vi "calc_sinlge JumpWaveform_v0.03.vi"(0 "New input cluster":T1={"Which Position to use for Experiment"=enum."Jumper Safe Position", "Start Position (N)"="", "Jump Position (m)"="", "Duration (s)"=0.0, "Delay (s)"=0.0, "Pulse Width (s)"=0.0, "Valve 1 Position"=0, "Valve 2 Position"=0, "Replicates"=0.0, "Vholding (mV)"=0.0, "Valve 3 Position"=1, "valve 1 used now?"=TRUE, "valve 2 used now?"=FALSE, "valve 3 used now? "=FALSE, "protocol Preview"=[]} {"Valve 3 Position" min=1 max=8}, 1 "Clear Waveform?":bool, 5 "Old input cluster":T1={"Which Position to use for Experiment"=enum."Jumper Safe Position", "Start Position (N)"="", "Jump Position (m)"="", "Duration (s)"=0.0, "Delay (s)"=0.0, "Pulse Width (s)"=0.0, "Valve 1 Position"=0, "Valve 2 Position"=0, "Replicates"=0.0, "Vholding (mV)"=0.0, "Valve 3 Position"=1, "valve 1 used now?"=TRUE, "valve 2 used now?"=FALSE, "valve 3 used now? "=FALSE, "protocol Preview"=[]} {"Valve 3 Position" min=1 max=8}, 7 "sample freq":i32=10000, 9 "Jump Filter Freq (Hz)":dbl=30.0, 11 "error in":errorcluster) -> (4 "output cluster":T1={"Which Position to use for Experiment"=enum."Jumper Safe Position", "Start Position (N)"="", "Jump Position (m)"="", "Duration (s)"=0.0, "Delay (s)"=0.0, "Pulse Width (s)"=0.0, "Valve 1 Position"=0, "Valve 2 Position"=0, "Replicates"=0.0, "Vholding (mV)"=0.0, "Valve 3 Position"=1, "valve 1 used now?"=TRUE, "valve 2 used now?"=FALSE, "valve 3 used now? "=FALSE, "protocol Preview"=[]} {"Valve 3 Position" min=1 max=8}, 15 "error out":errorcluster)   [LabVIEW 2019]
uses:
  <vilib>/Analysis/3filter.llb/Filter Passband Type.ctl
  <vilib>/Analysis/3filter.llb/Bessel Filter (DBL).vi
  <vilib>/Analysis/NI_AALBase.lvlib
  <vilib>/measure/NI_MABase.lvlib
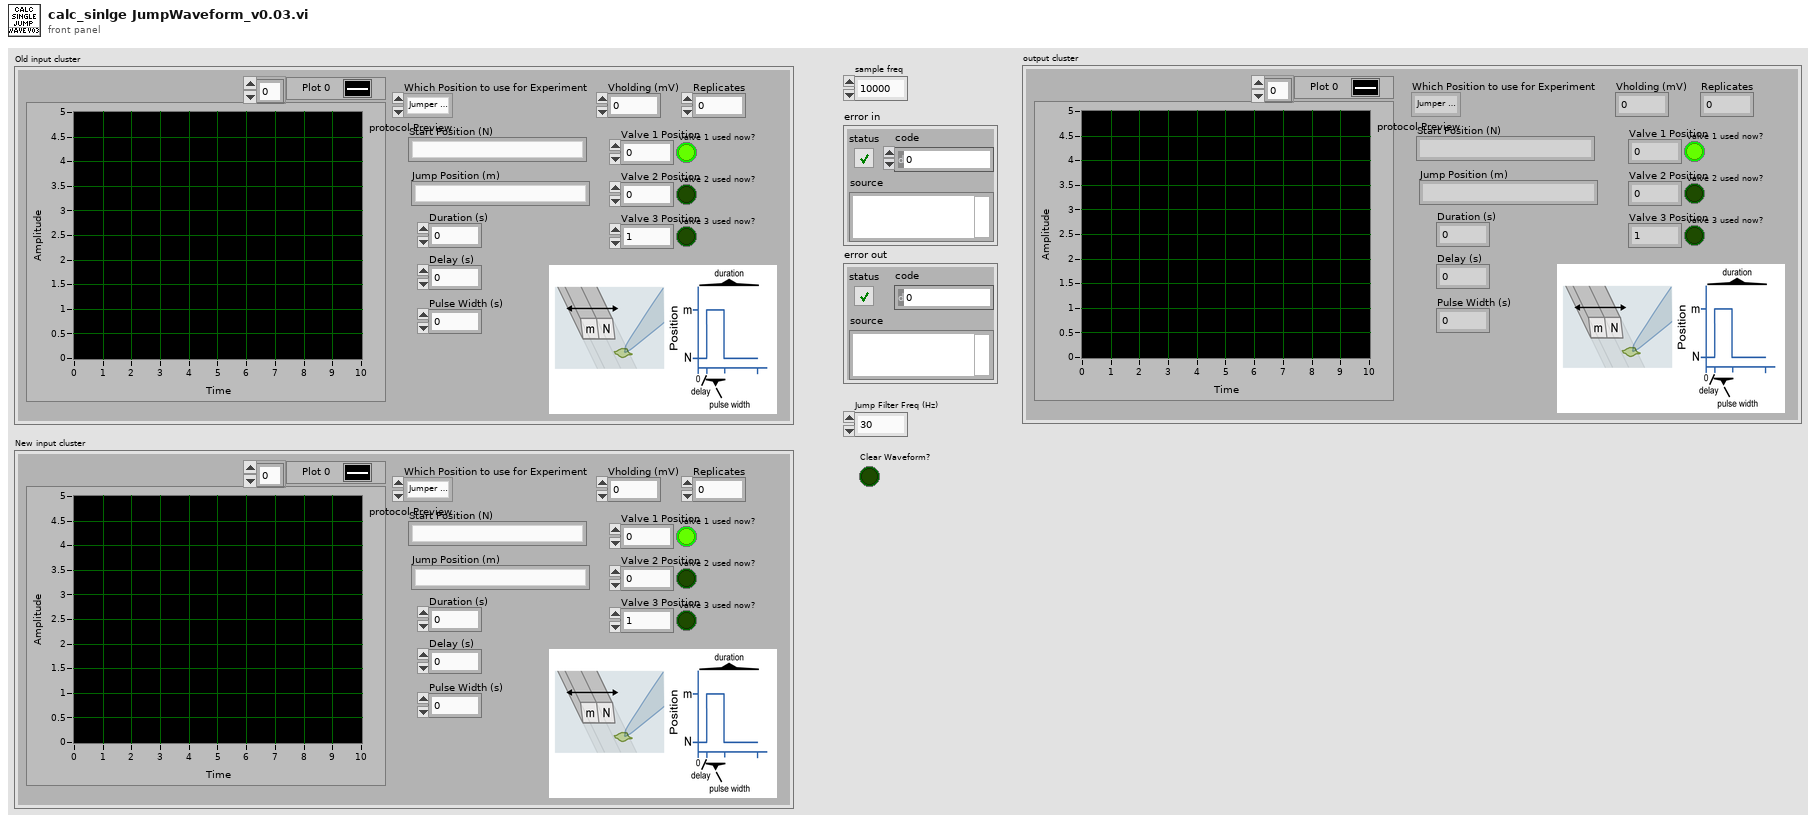
[diagram p1: front panel]
types:
  T1 = cluster{"Which Position to use for Experiment":enum16{"Jumper Safe Position", "Experiment Safe Position", "Jumper Position A", "Jumper Position B", "Jumper Position C", "Jumper Position o-A", "Jumper Position A-o", "Jumper Position A-B", "Jumper Position B-A", "Jumper Position B-C", "Jumper Position C-B", "Jumper Position C-o", "Jumper Position o-C", "Don't Move"}, "Start Position (N)":string, "Jump Position (m)":string, "Duration (s)":dbl, "Delay (s)":dbl, "Pulse Width (s)":dbl, "Valve 1 Position":i16, "Valve 2 Position":i16, "Replicates":dbl, "Vholding (mV)":dbl, "Valve 3 Position":i16, "valve 1 used now?":bool, "valve 2 used now?":bool, "valve 3 used now? ":bool, "protocol Preview":waveform(dbl)[]}
  T2 = enum16{"Jumper Safe Position", "Experiment Safe Position", "Jumper Position A", "Jumper Position B", "Jumper Position C", "Jumper Position o-A", "Jumper Position A-o", "Jumper Position A-B", "Jumper Position B-A", "Jumper Position B-C", "Jumper Position C-B", "Jumper Position C-o", "Jumper Position o-C", "Don't Move"}
  T3 = typedef "NI_AALBase.lvlib/Filter Passband Type.ctl" = enum32{"Lowpass", "Highpass", "Bandpass", "Bandstop"}
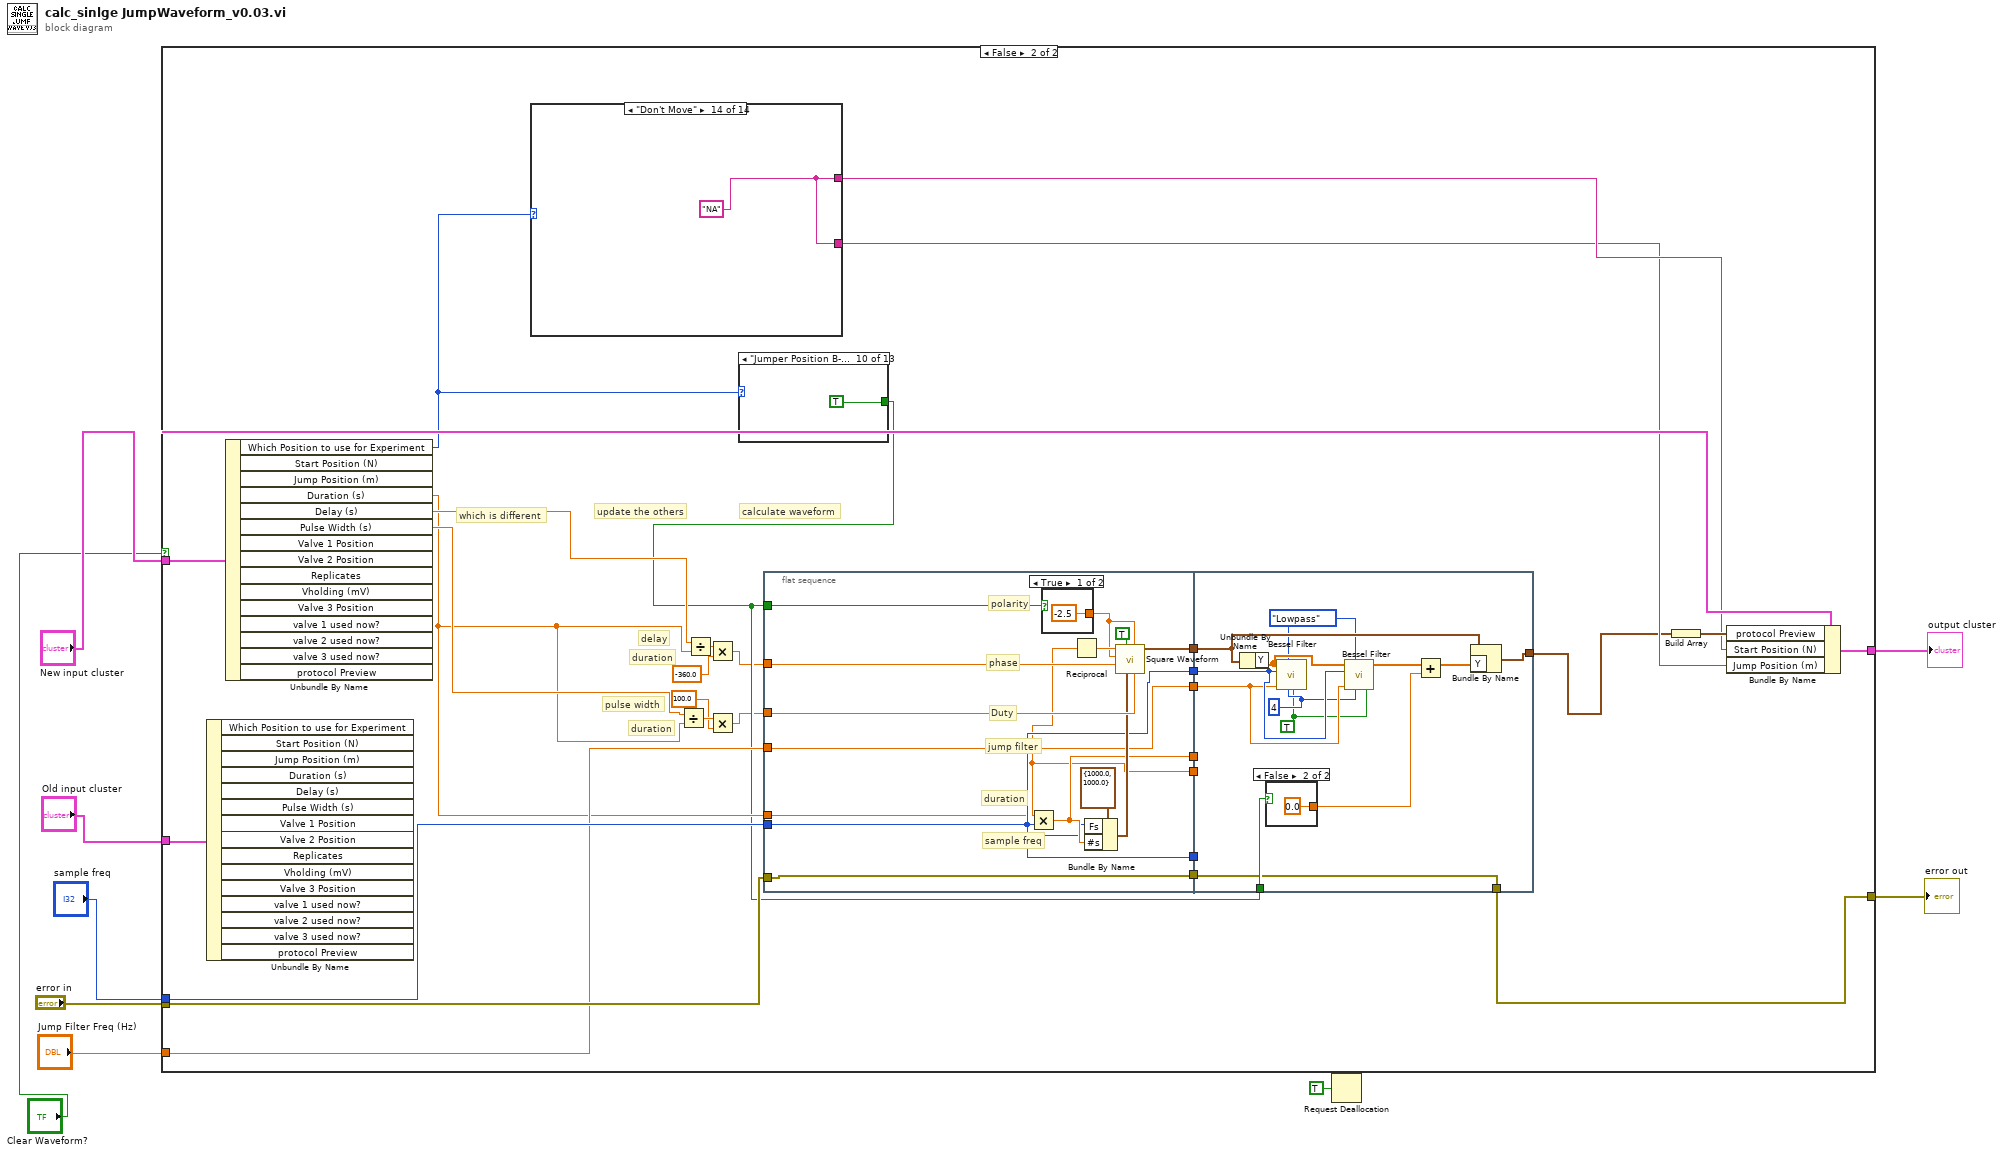
[diagram p0: block diagram]
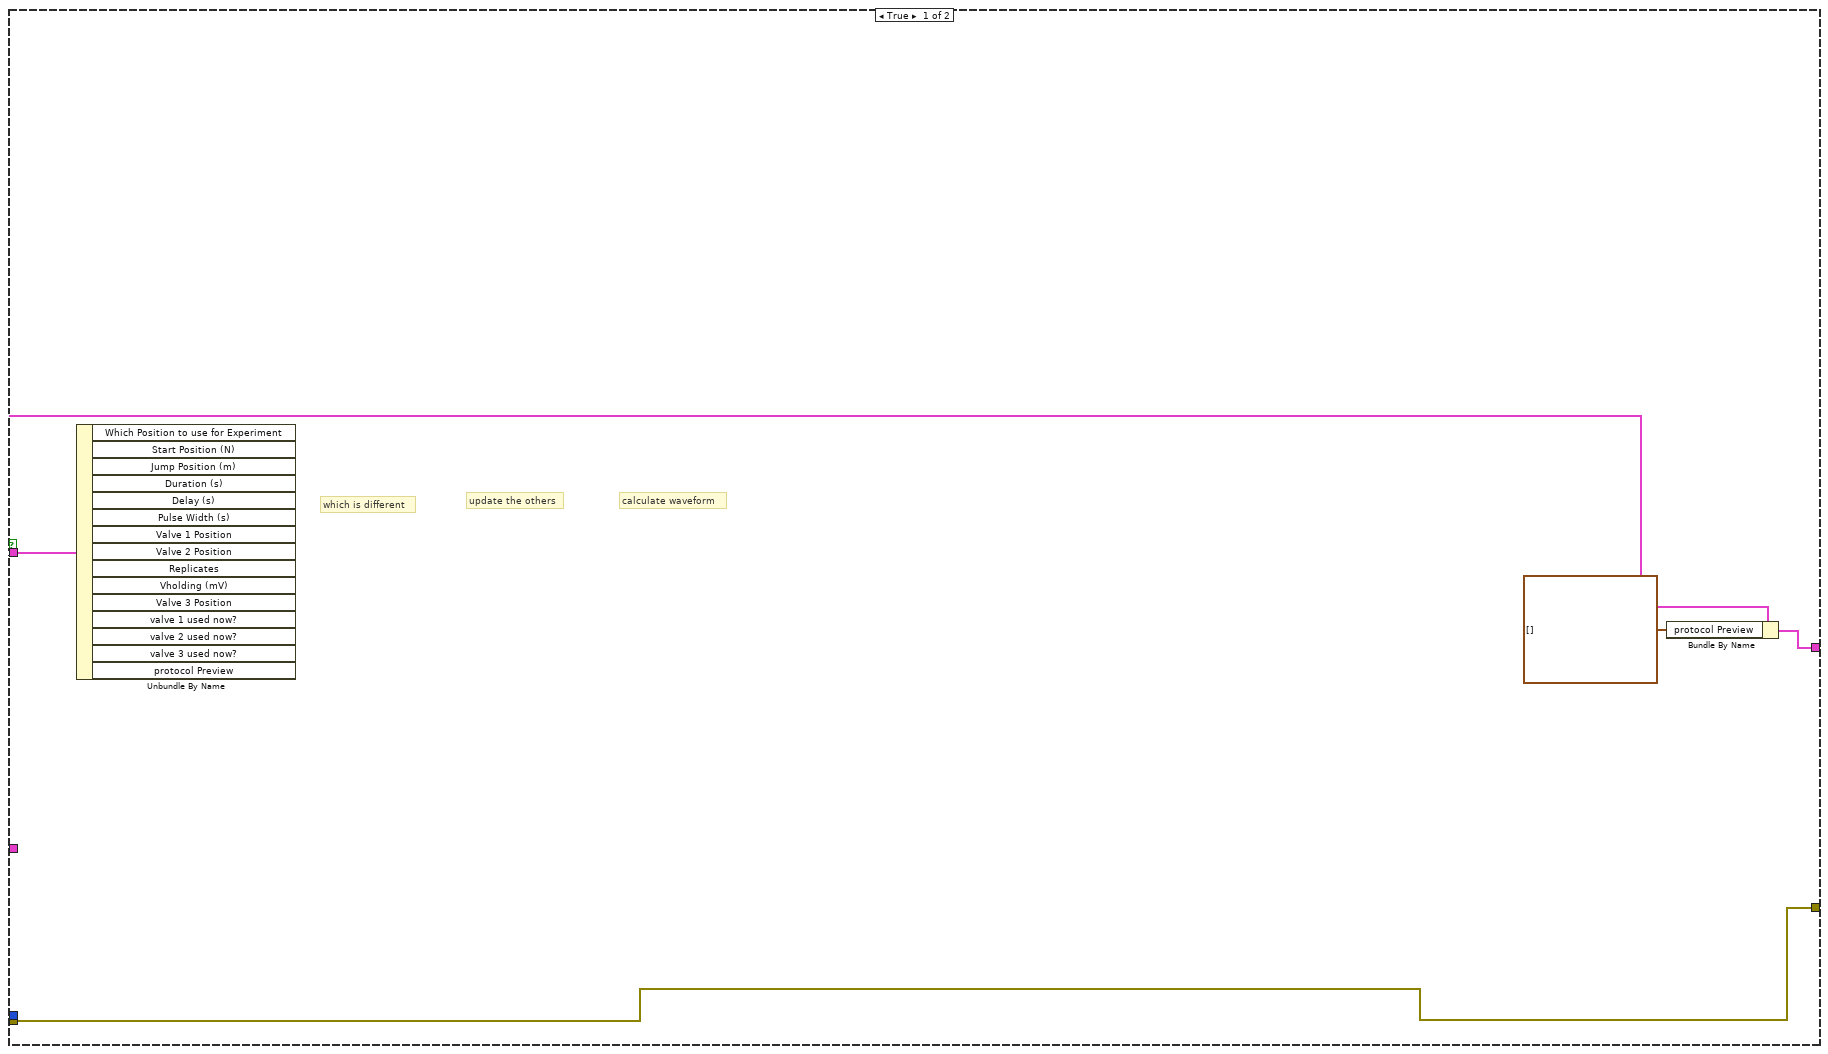
[diagram p2: hidden frame]
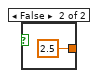
[diagram p3: hidden frame]
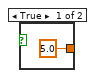
[diagram p4: hidden frame]
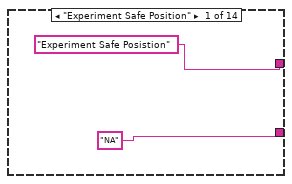
[diagram p5: hidden frame]
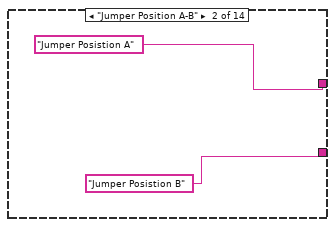
[diagram p6: hidden frame]
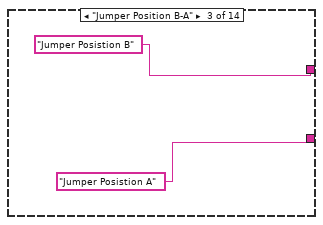
[diagram p7: hidden frame]
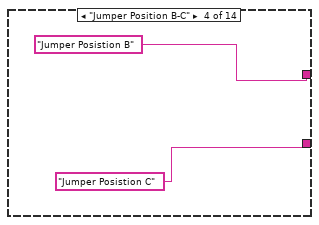
[diagram p8: hidden frame]
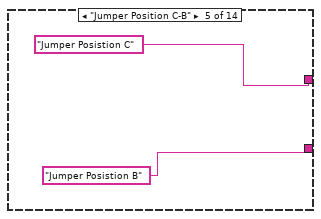
[diagram p9: hidden frame]
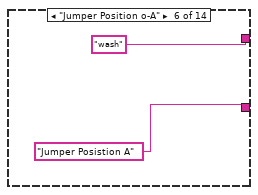
[diagram p10: hidden frame]
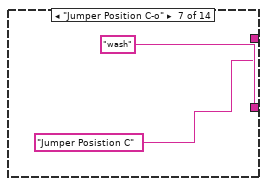
[diagram p11: hidden frame]
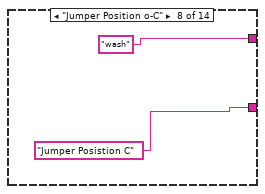
[diagram p12: hidden frame]
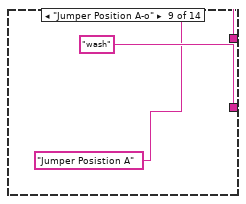
[diagram p13: hidden frame]
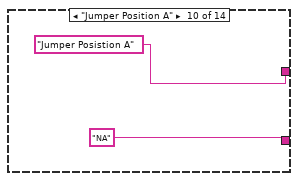
[diagram p14: hidden frame]
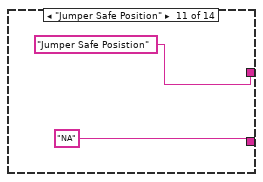
[diagram p15: hidden frame]
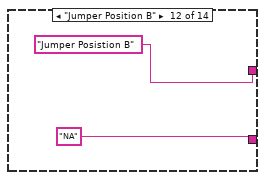
[diagram p16: hidden frame]
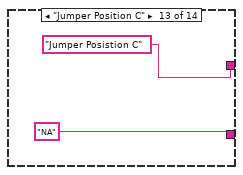
[diagram p17: hidden frame]
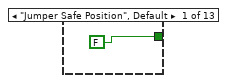
[diagram p18: hidden frame]
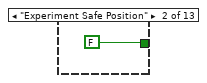
[diagram p19: hidden frame]
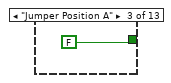
[diagram p20: hidden frame]
diagram:
  n1 = case shown="False" "Clear Waveform?" {
    tunnel: "New input cluster" -> [w13 w35]
    tunnel: [w12 w34] -> w8
    tunnel: "Old input cluster" -> [_ w33]
    tunnel: "error in" -> [w11 w28]
    tunnel: "sample freq" -> [_ w27]
    tunnel: "Jump Filter Freq (Hz)" -> [_ w26]
    tunnel: [w11 w21] -> w3
    frame True {
      # "calculate waveform"
      # "update the others"
      # "which is different"
      n2 = Unbundle By Name(w13) -> ()  [unwired: 15 out]
      n3 = Bundle By Name(cluster=w13, "protocol Preview"=waveform(dbl)[] []) -> (w12:T1)
    }
    frame False {
      # "pulse width"
      # "duration"
      # "duration"
      # "delay"
      # "calculate waveform"
      # "update the others"
      # "which is different"
      n4 = Unbundle By Name(w33) -> ()  [unwired: 15 out]
      n5 = Unbundle By Name(w35) -> ("Which Position to use for Experiment"=w31:T2, "Duration (s)"=w23:dbl, "Delay (s)"=w24:dbl, "Pulse Width (s)"=w25:dbl)  [unwired: 11 out]
      n6 = case shown="\"Don't Move\"" w31 {
        tunnel: ["Experiment Safe Posistion" "Jumper Posistion A" "Jumper Posistion B" "Jumper Posistion B" "Jumper Posistion C" "wash" "Jumper Posistion C" "wash" "Jumper Posistion A" "Jumper Posistion A" "Jumper Safe Posistion" "Jumper Posistion B" "Jumper Posistion C" w100] -> w30
        tunnel: ["NA" "Jumper Posistion B" "Jumper Posistion A" "Jumper Posistion C" "Jumper Posistion B" "Jumper Posistion A" "wash" "Jumper Posistion C" "wash" "NA" "NA" "NA" "NA" w100] -> w29
        frame "Experiment Safe Position" {
        }
        frame "Jumper Position A-B" {
        }
        frame "Jumper Position B-A" {
        }
        frame "Jumper Position B-C" {
        }
        frame "Jumper Position C-B" {
        }
        frame "Jumper Position o-A" {
        }
        frame "Jumper Position C-o" {
        }
        frame "Jumper Position o-C" {
        }
        frame "Jumper Position A-o" {
        }
        frame "Jumper Position A" {
        }
        frame "Jumper Safe Position" {
        }
        frame "Jumper Position B" {
        }
        frame "Jumper Position C" {
        }
        frame "Don't Move" {
          w100 = "NA"
        }
      }
      n7 = Divide(x=w25, y=w23) -> (x/y=w16:dbl)
      n8 = Divide(x=w24, y=w23) -> (x/y=w19:dbl)
      n9 = Multiply(x=w19, y=-360.0) -> (x*y=w17:dbl)
      n10 = Multiply(x=w16, y=100.0) -> (x*y=w14:dbl)
      n11 = case shown="\"Jumper Position B-C\"" w31 {
        tunnel: [FALSE FALSE FALSE FALSE FALSE TRUE FALSE TRUE FALSE TRUE FALSE TRUE FALSE] -> w22
        frame "Jumper Safe Position", Default {
        }
        frame "Experiment Safe Position" {
        }
        frame "Jumper Position A" {
        }
        frame "Jumper Position B" {
        }
        frame "Jumper Position C" {
        }
        frame "Jumper Position o-A" {
        }
        frame "Jumper Position A-o" {
        }
        frame "Jumper Position A-B" {
        }
        frame "Jumper Position B-A" {
        }
        frame "Jumper Position B-C" {
        }
        frame "Jumper Position C-B" {
        }
        frame "Jumper Position C-o" {
        }
        frame "Jumper Position o-C" {
        }
      }
      n12 = flat-sequence {
        tunnel: w17 -> [w56]
        tunnel: w14 -> [w55]
        tunnel: w23 -> [w43]
        tunnel: w26 -> [w50]
        tunnel: w27 -> [w49]
        tunnel: [w51] -> w42
        tunnel: [w49] -> w41
        tunnel: [w50] -> w40
        tunnel: [w49] -> w39
        tunnel: [w48] -> w38
        tunnel: w28 -> [w46]
        tunnel: [w46] -> w37
        tunnel: w22 -> [w45]
        tunnel: [w43] -> w36
        tunnel: w42 -> [_]
        tunnel: w41 -> [_]
        tunnel: w40 -> [w65]
        tunnel: w39 -> [w66]
        tunnel: w38 -> [w71]
        tunnel: w37 -> [w60]
        tunnel: w22 -> [w68]
        tunnel: w36 -> [_]
        tunnel: [w60] -> w21
        tunnel: [w59] -> w20
        frame #0 {
          # "sample freq"
          # "duration"
          # "jump filter"
          # "Duty"
          # "phase"
          # "polarity"
          n13 = Multiply(x=w43, y=w49) -> (x*y=w51:dbl)
          n14 = case shown="True" w45 {
            tunnel: [-2.5 ("Amplitude") 2.5 ("Amplitude")] -> w44
            frame True {
            }
            frame False {
            }
          }
          n15 = Reciprocal(x=w43) -> (1/x=w47:dbl)
          n16 = Bundle By Name(cluster=cluster{"Fs":dbl, "#s":dbl} {"Fs"=1000.0, "#s"=1000.0} ("sampling info"), "Fs"=w49, "#s"=w51) -> (w52:cluster{"Fs":dbl, "#s":dbl})
          n17 = call <vilib>:"Square Waveform.vi"("duty cycle (%)"=w55, "offset"=w44, "sampling info"=w52, "reset signal"=TRUE, "phase"=w56, "amplitude"=w44, "frequency"=w47) -> ("signal out"=w48:waveform(dbl))  [unwired: 3 in, 1 out]
        }
        frame #1 {
          w63 = TRUE ("init/cont (init:F)")
          w64 = 4 ("order")
          w62 = Filter_Passband_Type."Lowpass" ("filter type")
          n18 = Unbundle By Name(w71) -> ("Y"=w67:dbl[])
          n19 = case shown="False" w68 {
            tunnel: [5.0 ("Amplitude") 0.0 ("Amplitude")] -> w69
            frame True {
            }
            frame False {
            }
          }
          n20 = call-poly <vilib>:"Bessel Filter.vi"("init/cont (init:F)"=w63, "order"=w64, "filter type"=w62, "low cutoff freq: fl"=w65, "sampling freq: fs"=w66, "X"=w67) -> ()  [unwired: 2 in, 2 out]
          n21 = call-poly <vilib>:"Bessel Filter.vi"("init/cont (init:F)"=w63, "order"=w64, "filter type"=w62, "low cutoff freq: fl"=w65, "sampling freq: fs"=w66, "X"=w67) -> ("Filtered X"=w61:dbl[])  [unwired: 2 in, 1 out]
          n22 = Add(x=w61, y=w69) -> (x+y=w70:dbl[])
          n23 = Bundle By Name(cluster=w71, "Y"=w70) -> (w59:waveform(dbl))
        }
      }
      n24 = Build Array(w20) -> (w32:waveform(dbl)[])
      n25 = Bundle By Name(cluster=w35, "protocol Preview"=w32, "Start Position (N)"=w30, "Jump Position (m)"=w29) -> (w34:T1)
    }
  }
  "output cluster" <- w8
  "error out" <- w3
  n26 = Request Deallocation(TRUE ("flag")) -> ()
